vi "Is Triggered.vi"(8 "error in (no error)":errorcluster, 11 "Pulse Controller in":refnum<class "Pulse Recorder.lvclass">) -> (0 "error out":errorcluster, 2 "Triggered":bool, 3 "Pulse Controller out":refnum<class "Pulse Recorder.lvclass">)   [LabVIEW 2015, in "Pulse Recorder.lvclass"]
uses:
  Pulse Recorder.lvclass
  Pulse Recorder.lvclass/Pulse Recorder.ctl
  NHMFL_Core/Libraries/Instruments/Pulse Driver/Pulse Driver.lvclass
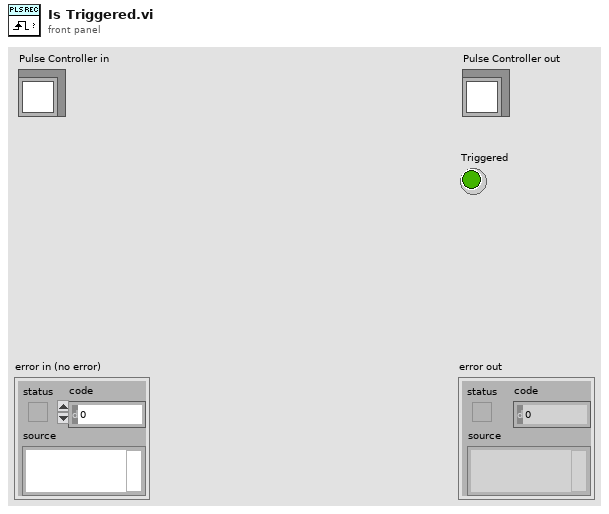
[diagram p1: front panel]
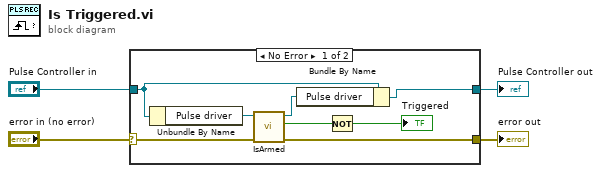
[diagram p0: block diagram]
diagram:
  n1 = case shown="No Error" "error in (no error)" {
    selector: "error in (no error)" -> [w7 w14]
    tunnel: [w6 w14] -> w3
    tunnel: [w8 w13] -> w1
    tunnel: "Pulse Controller in" -> [w9 w13]
    frame No Error {
      n2 = Unbundle By Name(w9) -> ("Pulse driver"=w10:refnum<class "Pulse Driver.lvclass">)
      n3 = call-dynamic "IsArmed.vi"("error in (no error)"=w7, "DAQmx Digitizer in"=w10) -> ("error out"=w6:errorcluster, "Armed"=w12:bool, "DAQmx Digitizer out"=w11:refnum<class "Pulse Driver.lvclass">)  [unwired: 5 in, 2 out]
      n4 = Bundle By Name(cluster=w9, "Pulse driver"=w11) -> (w8:refnum<class "Pulse Recorder.lvclass">)
      n5 = Not(x=w12) -> (.not. x?=→"Triggered":bool)
    }
    frame Error {
    }
  }
  "error out" <- w3
  "Pulse Controller out" <- w1
